vi "Get Best Path.vi"(8 "error in (no error)":errorcluster, 11 "TSP Class in":refnum<class "TSP Class.lvclass">) -> (0 "error out":errorcluster, 1 "Coordinate[]":T1[](array[typedef])=[{"x"=67.57906304229073, "y"=68.60831518225434}, {"x"=81.83522625397705, "y"=7.983158550148239}, {"x"=13.845000200345314, "y"=50.20462870854803}, {"x"=65.60632392598347, "y"=23.41592963463568}, {"x"=37.527186631799125, "y"=49.26560940206024}, {"x"=75.80408834272797, "y"=82.83507884873025}, {"x"=91.24590880296392, "y"=43.00621931342281}, {"x"=88.66715419959786, "y"=61.38804665807669}, {"x"=86.51526432096372, "y"=8.714647141634234}, {"x"=83.91892871742184, "y"=30.341190073224354}, {"x"=24.743038312024, "y"=79.88068424696041}, {"x"=25.30168704115323, "y"=47.03932115592622}, {"x"=88.22800157317587, "y"=11.43101038338128}], 2 "Distance":dbl, 3 "TSP Class out":refnum<class "TSP Class.lvclass">)   [LabVIEW 2015, in "TSP Library.lvlib" / "TSP Class.lvclass"]
uses:
  TSP Class.lvclass
  TypeDef/Coordinate.ctl
  TSP Class.lvclass/TSP Class.ctl
  TSP Library.lvlib
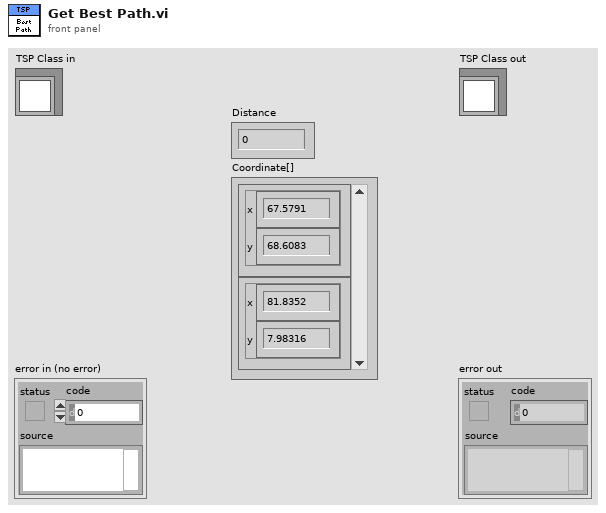
[diagram p1: front panel]
types:
  T1 = typedef "TSP Library.lvlib/Coordinate.ctl" = cluster{"x":dbl, "y":dbl}
  T2 = typedef "TSP Library.lvlib/Path.ctl" = cluster{"Distance":dbl, "Coordinate[]":T1[]}
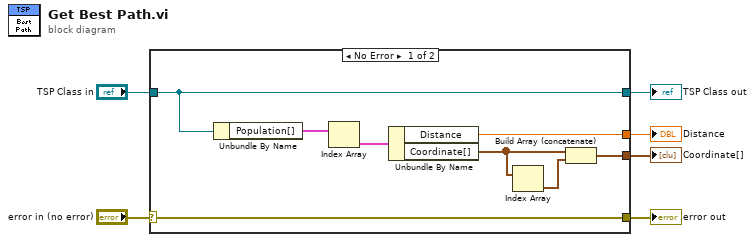
[diagram p0: block diagram]
diagram:
  n1 = case shown="No Error" "error in (no error)" {
    selector: "error in (no error)" -> [w14 w16]
    tunnel: [w14 w16] -> w5
    tunnel: [w13 w15] -> w3
    tunnel: "TSP Class in" -> [w13 w15]
    tunnel: [w8 _] -> w2
    tunnel: [w7 _] -> w1
    frame No Error {
      n2 = Unbundle By Name(w13) -> ("Population[]"=w12:T2[])
      n3 = Index Array(array=w12) -> (element=w9:T2)  [unwired: 1 in]
      n4 = Unbundle By Name(w9) -> ("Distance"=w8:dbl, "Coordinate[]"=w11:T1[])
      n5 = Index Array(array=w11) -> (element=w10:T1)  [unwired: 1 in]
      n6 = Build Array (concatenate)(w11, w10) -> (w7:T1[])
    }
    frame Error {
    }
  }
  "error out" <- w5
  "TSP Class out" <- w3
  "Distance" <- w2
  "Coordinate[]" <- w1
